vi "NI update wav display.vi"(8 "error in (no error)":errorcluster, 11 "NI in":refnum<class "NI.lvclass">) -> (0 "error out":errorcluster, 3 "NI out":refnum<class "NI.lvclass">)   [LabVIEW 2021, in "NI.lvlib" / "NI.lvclass"]
uses:
  NI.lvclass
  NI.lvclass/NI.ctl
  <vilib>/DAQmx/read.llb/DAQmx Read (Analog 1D DBL 1Chan NSamp).vi
  <vilib>/DAQmx/miscellaneous.llb/DAQmx Fill In Error Info.vi
  <resource>/objmgr/daqmx.rc
panel:
  in  "num samples":i32=5000
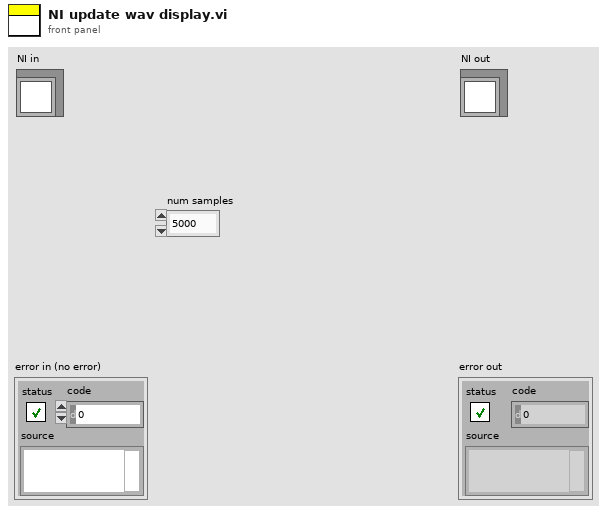
[diagram p1: front panel]
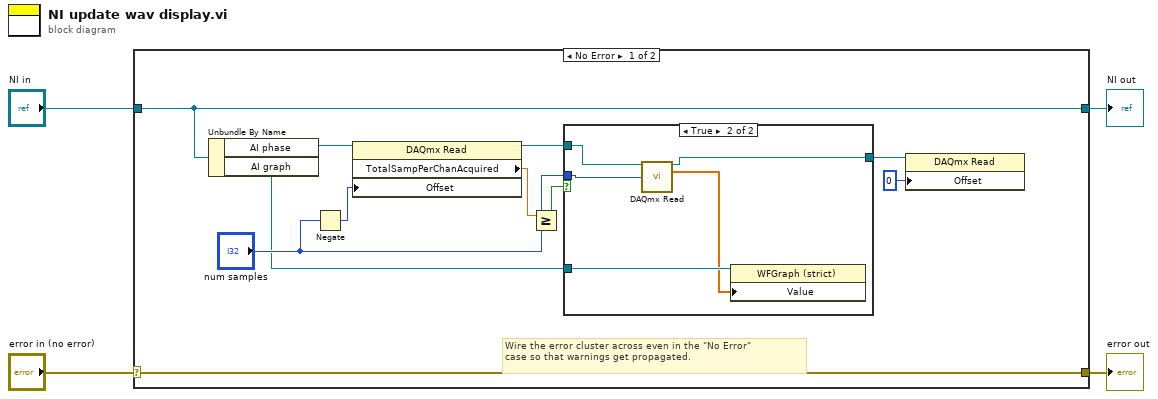
[diagram p0: block diagram]
diagram:
  n1 = case shown="No Error" "error in (no error)" {
    selector: "error in (no error)" -> [w15 w23]
    tunnel: [w15 w23] -> w3
    tunnel: [w14 w22] -> w1
    tunnel: "NI in" -> [w14 w22]
    frame No Error {
      # "Wire the error cluster across even in the \"No Error\"\ncase so that warnings get propagated."
      n2 = Unbundle By Name(w14) -> ("AI phase"=w13:refnum<k21>, "AI graph"=w5:refnum<vi>)
      n3 = Negate(x="num samples") -> (-x=w7:i32)
      n4 = property class="DAQmx Read"(reference=w13, "Offset"=w7) -> (reference out=w12:refnum<k21>, "TotalSampPerChanAcquired"=w10:dbl)  [unwired: 1 in, 1 out]
      n5 = Greater Or Equal?(x=w10, y="num samples") -> (x >= y?=w9:bool)
      n6 = case shown="True" w9 {
        tunnel: w12 -> [w16 w21]
        tunnel: [w16 w20] -> w11
        tunnel: "num samples" -> [_ w19]
        tunnel: w5 -> [_ w18]
        frame False {
        }
        frame True {
          n7 = call-poly <vilib>:"DAQmx Read.vi"("task/channels in"=w21, "number of samples per channel"=w19) -> ("task out"=w20:refnum<k21>, "data"=w17:dbl[])  [unwired: 11 in, 1 out]
          n8 = property class="WFGraph (strict)"(reference=w18, "Value"=w17) -> ()  [unwired: 1 in, 2 out]
        }
      }
      n9 = property class="DAQmx Read"(reference=w11, "Offset"=0) -> ()  [unwired: 1 in, 2 out]
    }
    frame Error {
    }
  }
  "error out" <- w3
  "NI out" <- w1
